vi "sobre.vi"   [LabVIEW 2018]
panel:
  # "Gerador de Sinais"
  # "Especificações:"
  # "Freq. Máxima: 100 KHz\nFreq. de Aquisição: 1 MHz\nTensão: ± 10 Vp"
  # "Para obter ajuda, clique no botão '?'"
  # "Projeto de Estágio"
  # "Isabelle Orlandi"
  # "versão 1.0"
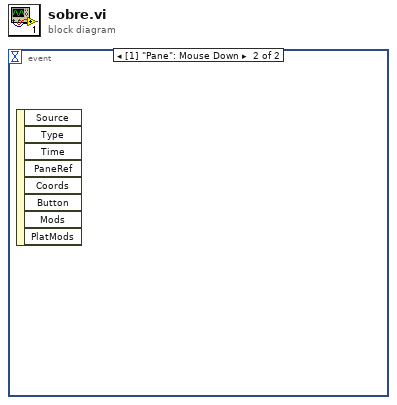
[diagram p0: block diagram]
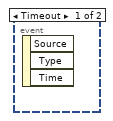
[diagram p2: hidden frame]
diagram:
  n1 = event shown="[1] \"Pane\": Mouse Down" {
    selector: _ -> [_ _]
    dyn-events: _ -> [_ _]
    timeout: _ -> [_ _]
    event Timeout {
      n2 = event-data() -> ()  [unwired: 1 in, 3 out]
    }
    event Mouse Down {
      n3 = event-data() -> ()  [unwired: 1 in, 8 out]
    }
  }
